vi "COMprompt.vi"(11 "Devices":string[](array[string])) -> (1 "Numeric":i32)   [LabVIEW 2012]
panel:
  in  "Select Device":i32(ring)=1 items=["WFT SynthNV 99", "WFT SynthNV 68"]
  in  "stop":bool
  # "Multiple SynthNVs Detected."
  # "Please select a Device."
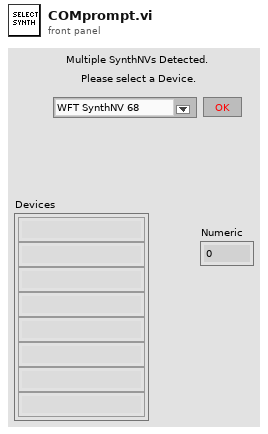
[diagram p1: front panel]
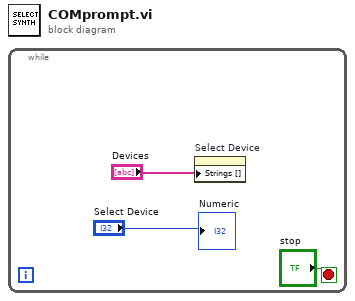
[diagram p0: block diagram]
diagram:
  n1 = while {
    stop <- "stop" stop-if-true
    n2 = property on="Select Device" class="Ring (strict)"("Strings []"="Devices") -> ()  [unwired: 2 in, 2 out]
    "Numeric" <- "Select Device"
  }
